vi "Right Variables.vi"() -> ()   [LabVIEW 2015]
panel:
  in  "R o2 X Center":u16
  in  "R o2 Y Center":u16
  in  "R o1 X Center":u16
  in  "R o1 Y Center":u16
  in  "RB Tracked?":bool
  in  "R Avg TB X Center":dbl
  in  "R Avg TB Y Center":dbl
  in  "R Raw TB X Center":u16
  in  "R Raw TB Y Center":u16
  in  "R Left Beacon Angle":dbl
  in  "R Right Beacon Angle":dbl
  in  "R Tilt Pulse Width":u32
  in  "R Run Tilt Motor":bool
  in  "R Unknown Beacon Angle 1":dbl
  in  "R Unknown Beacon Angle 2":dbl
  in  "R Data Valid?":bool
  in  "R Pan Pulse Width":u32
  in  "R Run Pan Motor":bool
  in  "R Y Avg":bool
  in  "R X Avg":bool
  in  "R Avg RB X Center":dbl
  in  "R Avg RB Y Center":dbl
  in  "R Avg LB X Center":dbl
  in  "R Avg LB Y Center":dbl
  in  "R STOP":bool
  in  "R Avg Distance (ft)":dbl
  in  "RT Stable":bool
  in  "RP Stable":bool
  in  "RT Limit Reached":bool
  in  "R State":string
  in  "R Avg Zone":dbl
  in  "R Raw RB X Center":u16
  in  "R Raw RB Y Center":u16
  in  "R Raw LB X Center":u16
  in  "R Raw LB Y Center":u16
  in  "RP Limit Reached":bool
  in  "R Dec Speed Zone":dbl
  in  "R Pan Angle":dbl
  in  "R Tilt Angle":dbl
  in  "R Pan Direction":bool
  in  "R Tilt Direction":bool
  in  "R Distance (in)":dbl
  in  "R Distance (ft)":dbl
  in  "R Distance (cm)":dbl
  in  "R Tilt Upper Limit":u16
  in  "R Tilt Lower Limit":u16
  in  "R Pan Upper Limit":u16
  in  "R Pan Lower Limit":u16
  in  "R Default Pulse Width":u32
  in  "R Pan Count":i32
  in  "R Tilt Count":i32
  # "RAW + AVG\nLIDAR\nData"
  # "AVG\nBeacon\n( X , Y )"
  # "TRACKED\nBeacon\n( X , Y )"
  # "o1\no2\n( X , Y )"
  # "RAW\nBeacon\n( X , Y )"
  # "Motor\nStep\nCounts"
  # "Motor\nPosition\nAngles"
  # "Unknown\nBeacon\nAngles"
  # "Deduced\nBeacon\nAngles"
  # "Tracking\nDead Zone\nLimits"
  # "Special\nTracking Zone\nDomains"
  # "Motor\nPulse\nWidths"
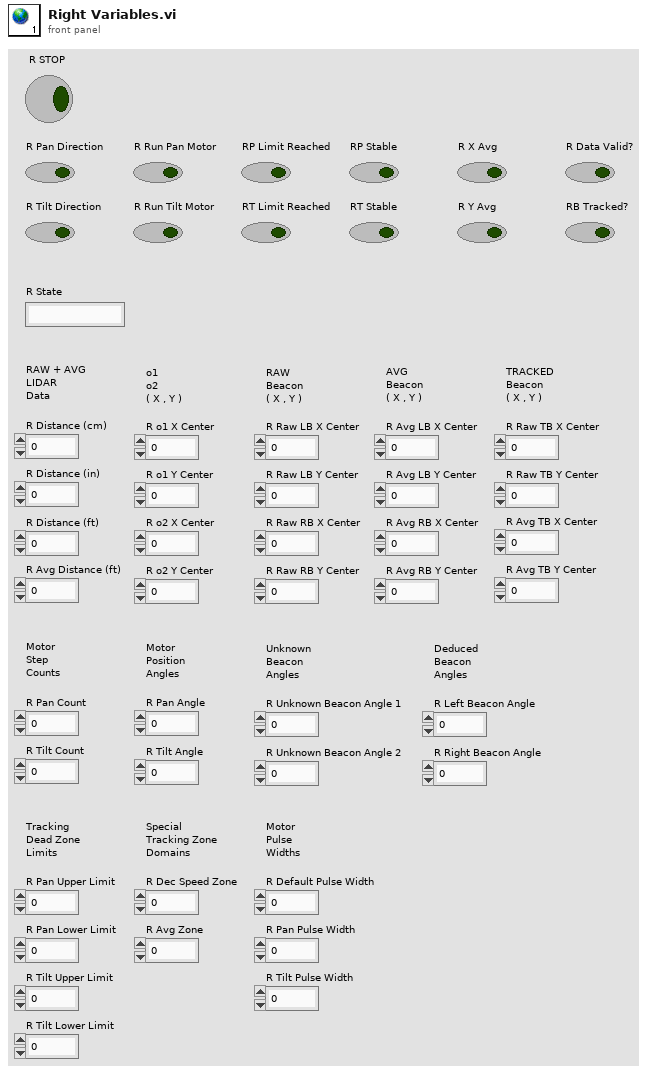
[diagram p1: front panel]
diagram:
